vi "Create Pattern Script - Rd Collect Frame.vi"(8 "error in (no error)":errorcluster, 11 "BML Pattern Creater.lvclass":refnum<class "BML Pattern Creater.lvclass">) -> (0 "error out":errorcluster, 2 "Rd Collect out":string, 3 "BML Pattern Creater.lvclass":refnum<class "BML Pattern Creater.lvclass">)   [LabVIEW 2018, in "BML Pattern Creater.lvlib" / "BML Pattern Creater.lvclass"]
uses:
  BML Pattern Creater.lvclass
  Ctls/OM - BML.ctl
  Special Frame.ctl
  Ctls/RW Options.ctl
  BML Pattern Creater.lvclass/BML Pattern Creater.ctl
  Write BML OM.vi
  Write R_W_.vi
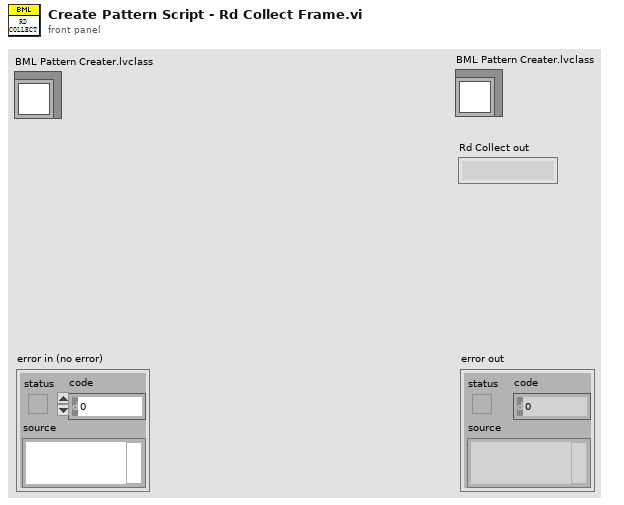
[diagram p1: front panel]
types:
  T1 = typedef "RW Options.ctl" = enum16{"Read", "Write", "R/W"}
  T2 = typedef "BML Pattern Creater.lvlib/BML Pattern Creater.lvclass/Special Frame.ctl" = enum16{"Sync Header", "BML Header", "SW Trig", "SetID State", "Exit SetID State", "SW Reset", "Wait"}
  T3 = typedef "OM - BML.ctl" = enum16{"Normal", "ImmeEffect", "InitSlaveID", "LoadData"}
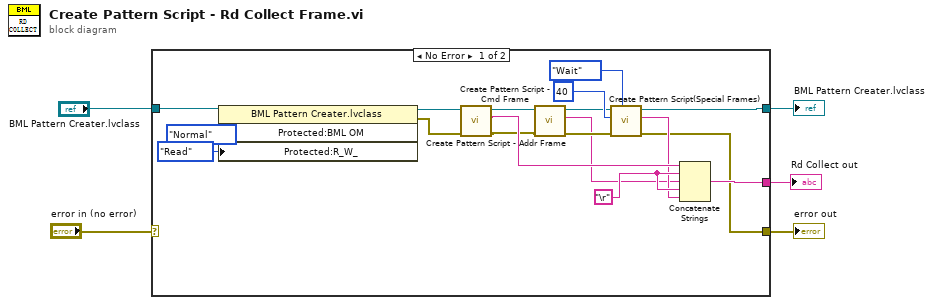
[diagram p0: block diagram]
diagram:
  n1 = case shown="No Error" "error in (no error)" {
    selector: "error in (no error)" -> [_ w25]
    tunnel: [w8 w25] -> w4
    tunnel: "BML Pattern Creater.lvclass" -> [w21 w24]
    tunnel: [w23 _] -> w3
    tunnel: [w7 w24] -> w1
    frame No Error {
      w22 = "\r"
      n2 = property class="BML Pattern Creater.lvclass"(reference=w21, "Protected:BML OM"=OM_-_BML."Normal" ("BML OM"), "Protected:R_W_"=RW_Options."Read" ("R_W_")) -> (reference out=w19:refnum<class "BML Pattern Creater.lvclass">, error out=w18:errorcluster)  [unwired: 1 in]
      n3 = call "Create Pattern Script - Cmd Frame.vi"("error in (no error)"=w18, "BML Pattern Creater in"=w19) -> ("error out"=w15:errorcluster, "CMD Frame out"=w17:string, "BML Pattern Creater out"=w16:refnum<class "BML Pattern Creater.lvclass">)  [unwired: 7 in]
      n4 = call "Create Pattern Script - Addr Frame.vi"("error in (no error)"=w15, "BML Pattern Creater in"=w16) -> ("error out"=w10:errorcluster, "Addr Frame"=w9:string, "BML Pattern Creater out"=w12:refnum<class "BML Pattern Creater.lvclass">)  [unwired: 7 in]
      n5 = call "Create Pattern Script(Special Frames).vi"("Special Frame Type"=Special_Frame."Wait", "error in (no error)"=w10, "Num of Timeset"=u32 40, "BML Pattern Creater in"=w12) -> ("error out"=w8:errorcluster, "string out"=w14:string, "BML Pattern Creater out"=w7:refnum<class "BML Pattern Creater.lvclass">)  [unwired: 5 in]
      n6 = Concatenate Strings(w17, w22, w9, w22, w14) -> (w23:string)
    }
    frame Error {
    }
  }
  "error out" <- w4
  "Rd Collect out" <- w3
  "BML Pattern Creater.lvclass" <- w1
